vi "Updated Command Status.vi"(8 "error in (no error)":errorcluster, 10 "Command Status":T1, 11 "System Actor in":refnum<class "System Actor.lvclass">) -> (0 "error out":errorcluster, 3 "System Actor out":refnum<class "System Actor.lvclass">)   [LabVIEW 2014, in "Robot Actor Framework.lvlib" / "System Actor.lvlib" / "System Actor.lvclass"]
uses:
  System Actor.lvclass
  Command Actor/Command Actor Class/Command State.ctl
  Command Actor/Command Actor Class/Command States.ctl
  Command Actor/Command Actor Class/Command Actor.lvclass
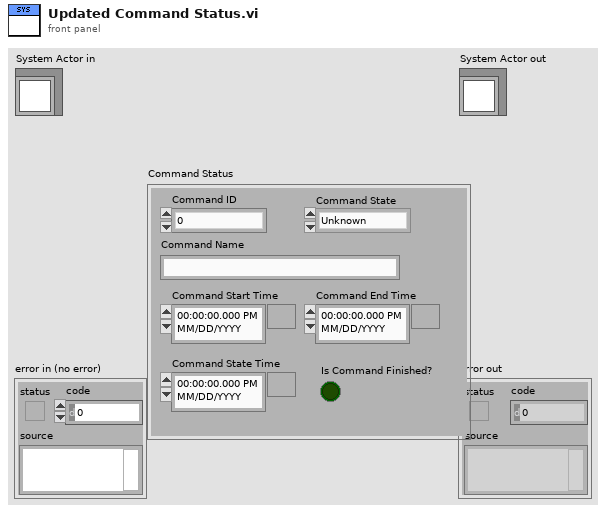
[diagram p1: front panel]
types:
  T1 = typedef "Robot Actor Framework.lvlib/Command Actor.lvlib/Command Actor.lvclass/Command State.ctl" = cluster{"Command Name":string, "Command Start Time":timestamp, "Command End Time":timestamp, "Is Command Finished?":bool, "Command ID":u32, "Command State":T2, "Command State Time":timestamp}
  T2 = typedef "Robot Actor Framework.lvlib/Command Actor.lvlib/Command Actor.lvclass/Command States.ctl" = enum16{"Unknown", "Started", "Stopped", "Finished"}
  T3 = typedef "Robot Actor Framework.lvlib/System Actor.lvlib/System Actor.lvclass/System State.ctl" = cluster{"Instance Name":string, "Current Command Status":T1, "System Start Time":timestamp, "Next Command ID":dbl, "Command Processor Status":T4}
  T4 = typedef "Robot Actor Framework.lvlib/Command Processor Actor.lvlib/Command Processor Actor.lvclass/Command Processor State.ctl" = cluster{"Current State":T5, "Last State Update":timestamp, "Queued Commands":u32, "Current Command Status":T1, "Previous State":T5, "Current State Entry":timestamp, "Transitioning State":bool, "Commands Behind":dbl, "Last Command Queue Time":timestamp}
  T5 = typedef "Robot Actor Framework.lvlib/Command Processor Actor.lvlib/Command Processor Actor.lvclass/Command Processor States.ctl" = enum16{"Unknown", "No Command", "Running Command", "Starting Command", "Stopping Command", "Finishing Command"}
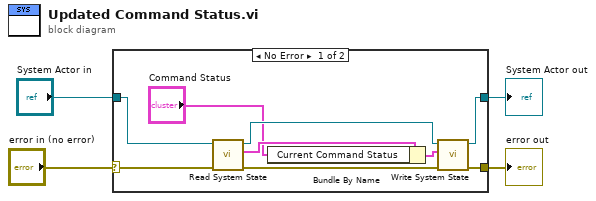
[diagram p0: block diagram]
diagram:
  n1 = case shown="No Error" "error in (no error)" {
    selector: "error in (no error)" -> [w7 w15]
    tunnel: [w5 w15] -> w3
    tunnel: [w8 w14] -> w1
    tunnel: "System Actor in" -> [w9 w14]
    frame No Error {
      n2 = call-dynamic "Read System State.vi"("error in (no error)"=w7, "System Actor in"=w9) -> ("error out"=w6:errorcluster, "System Status"=w12:T3, "System Actor out"=w13:refnum<class "System Actor.lvclass">)  [unwired: 7 in]
      n3 = Bundle By Name(cluster=w12, "Current Command Status"="Command Status") -> (w11:T3)
      n4 = call-dynamic "Write System State.vi"("error in (no error)"=w6, "System Status"=w11, "System Actor in"=w13) -> ("error out"=w5:errorcluster, "System Actor out"=w8:refnum<class "System Actor.lvclass">)  [unwired: 7 in]
    }
    frame Error {
    }
  }
  "error out" <- w3
  "System Actor out" <- w1
